vi "Create User Event - ConnectionEvent.vi"(8 "error in (no error)":errorcluster, 10 "ConnectionInfo":T1) -> (0 "error out":errorcluster, 3 "ConnectionEvent":refnum<user-event>)   [LabVIEW 2022 SP3, in "User Event - ConnectionEvent.lvlib"]
doc: "Create a boolean user event that will be used to stop the event loop from the message handling loop."
uses:
  User Event - ConnectionEvent.lvlib
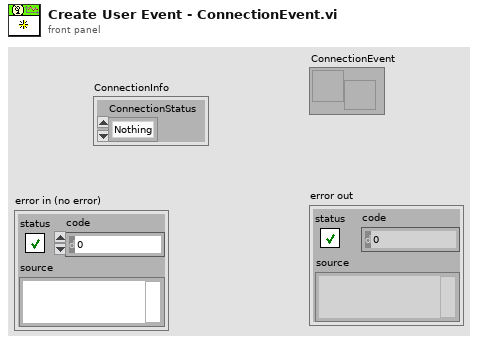
[diagram p1: front panel]
types:
  T1 = cluster{"ConnectionStatus":enum16{"Nothing", "Disconnect", "Connect", "Error"}}
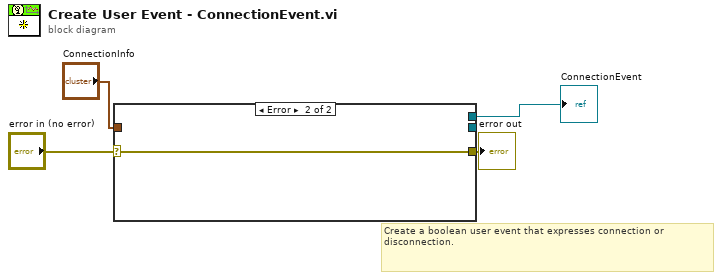
[diagram p0: block diagram]
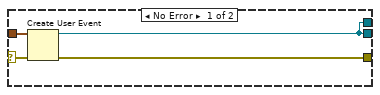
[diagram p2: hidden frame]
diagram:
  # "Create a boolean user event that expresses connection or disconnection."
  n1 = case shown="Error" "error in (no error)" {
    selector: "error in (no error)" -> [w7 w9]
    tunnel: [w8 w9] -> w4
    tunnel: "ConnectionInfo" -> [w6 _]
    tunnel: [w5 _] -> _
    tunnel: [w5 _] -> w1
    frame No Error {
      n2 = Create User Event(user event datatype=w6, error in=w7) -> (user event=w5:refnum<user-event>, error out=w8:errorcluster)
    }
    frame Error {
    }
  }
  "error out" <- w4
  "ConnectionEvent" <- w1
